vi "Serial_Close.vi"(8 "error in (no error)":errorcluster, 11 "Python in":T1) -> ()   [LabVIEW 2020]
uses:
  PythonCtrl.ctl
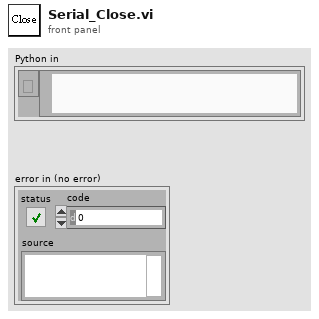
[diagram p1: front panel]
types:
  T1 = typedef "PythonCtrl.ctl" = cluster{"session":refnum<k35>, "PyPath":path}
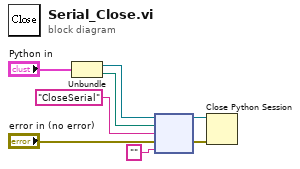
[diagram p0: block diagram]
diagram:
  n1 = Unbundle("Python in") -> ("session"=w7:refnum<k35>, "PyPath"=w8:path)
  n2 = node(w7, w8, "CloseSerial" ("function name"), "error in (no error)", "" ("function name")) -> (w2:refnum<k35>, w1:errorcluster)  [unwired: 1 in, 2 out]
  n3 = Close Python Session(session in=w2, error in=w1) -> ()  [unwired: 1 out]
